vi "CAN Read Engine.vi"(6 "Current Scoket":i16, 8 "error in (no error)":errorcluster, 9 "Selected Sockets":i16[](array[numeric]), 10 "CAN Ref Out":refnum<class "NI-XNET.lvclass">[](array[class]), 11 "Notifier in":refnum<notifier>) -> (0 "error out":errorcluster)   [LabVIEW 2023, in "LTT_TeststandSteptypes.lvlib"]
uses:
  LTT_TeststandSteptypes.lvlib
  HardwareAbstractionLayer_LVOOP/CAN/CAN Lib/NI-XNET_class/NI-XNET.lvclass
  HardwareAbstractionLayer_LVOOP/CAN/CAN Lib/Control/CAN Table.ctl
  <vilib>/xnet/xnet.llb/XNET Frame CAN.ctl
  <vilib>/xnet/xnet.llb/XNET Frame Type CAN.ctl
  Control/CAN FGV State.ctl
  HardwareAbstractionLayer_LVOOP/Database/Database.lvclass
  HardwareAbstractionLayer_LVOOP/CAN/CAN Lib/CAN HAL Lib.lvlib
panel:
  in  "CAN View Table":T1=-1
  out "Read":bool
  out "Send":bool
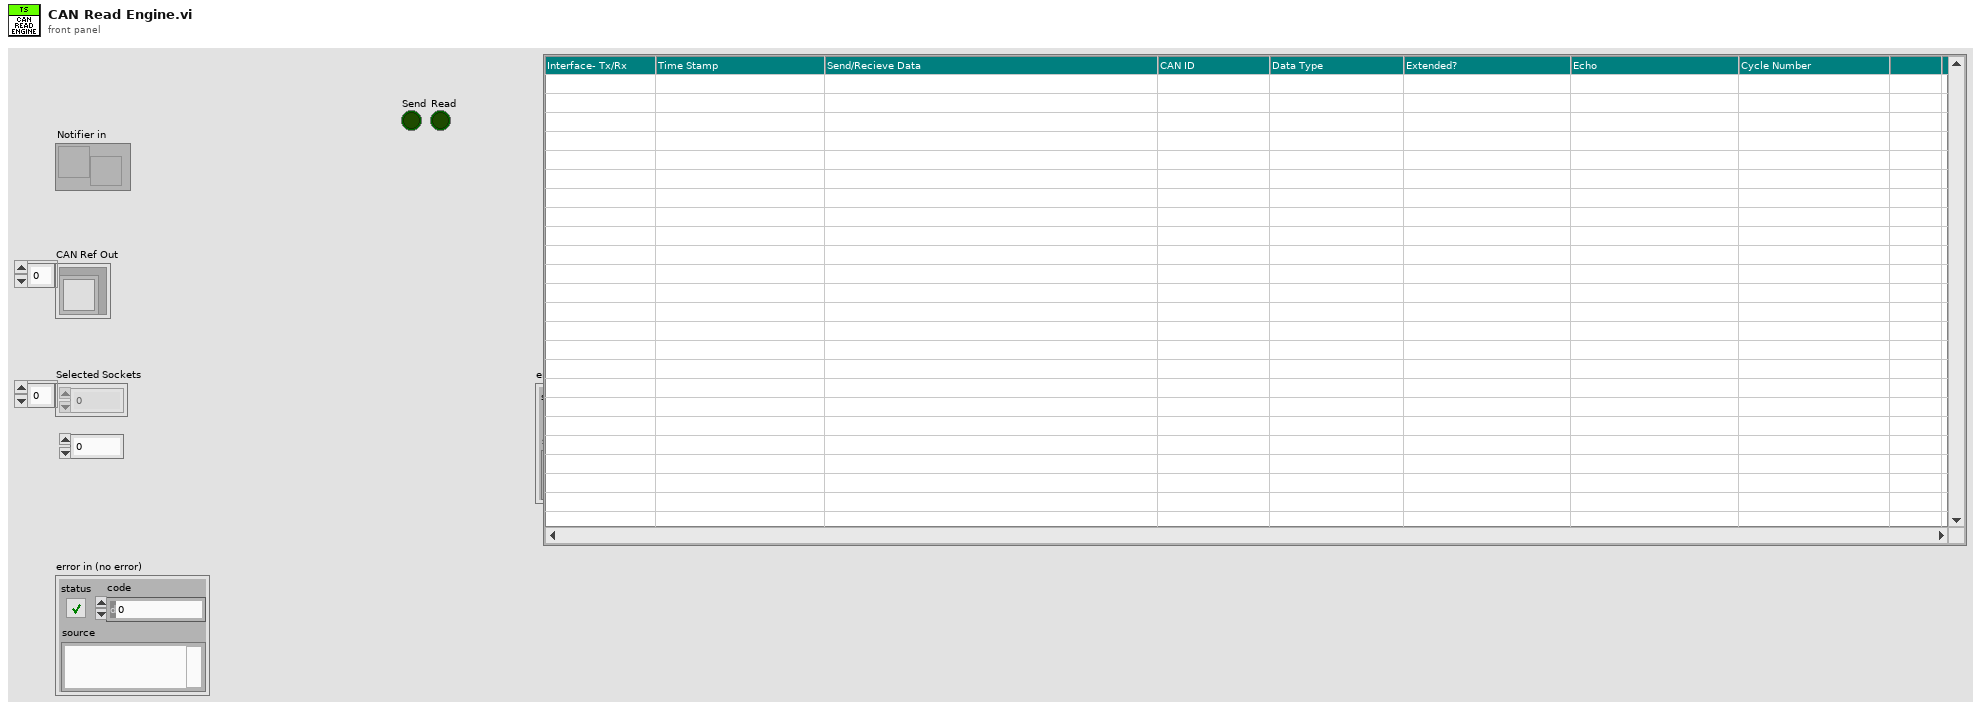
[diagram p1: front panel]
types:
  T1 = typedef "HardwareAbstractionLayer_LVOOP.lvlib/CAN HAL Lib.lvlib/CAN Table.ctl" = i32
  T2 = typedef "LTT_TeststandSteptypes.lvlib/CAN FGV State.ctl" = enum16{"Init", "Get", "Set"}
  T3 = typedef "XNET Frame CAN.ctl" = cluster{"timestamp":timestamp, "payload":u8[], "identifier":u32, "type":T4, "extended?":bool, "echo?":bool}
  T4 = typedef "XNET Frame Type CAN.ctl" = u8
  T5 = typedef "Semaphore RefNum" = refnum<k1>
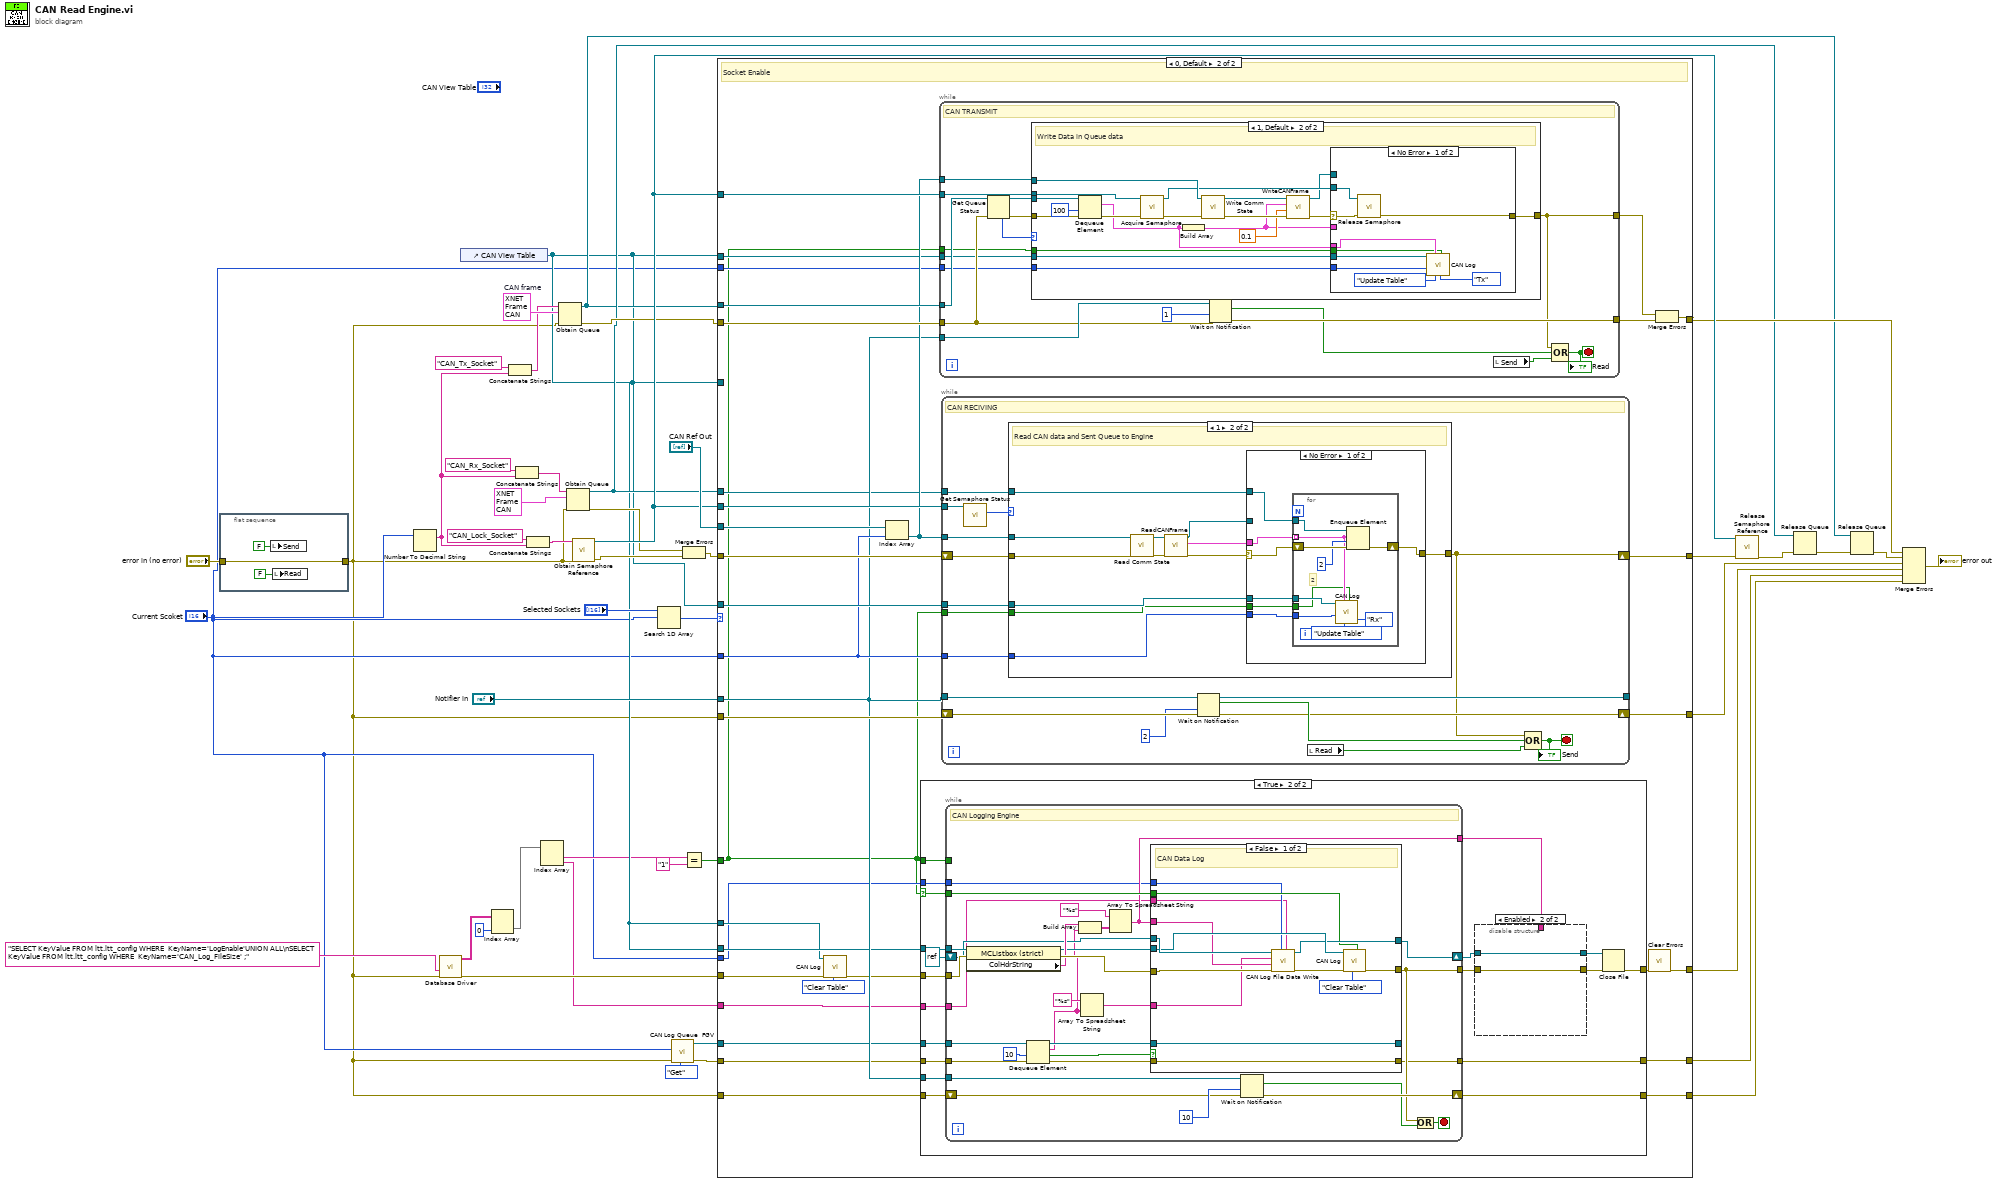
[diagram p0: block diagram]
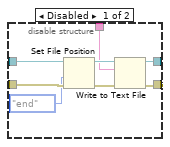
[diagram p4: hidden frame]
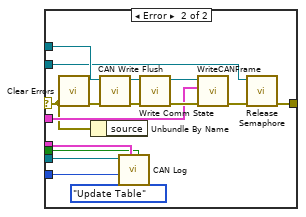
[diagram p7: hidden frame]
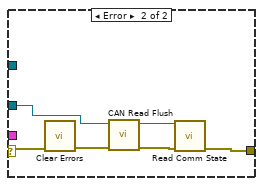
[diagram p9: hidden frame]
diagram:
  w35 = T3 {"timestamp"=timestamp(0 s since 1904-01-01), "payload"=[], "identifier"=0, "type"=0, "extended?"=FALSE, "echo?"=FALSE}  # CAN frame
  n1 = flat-sequence {
    tunnel: "error in (no error)" -> [w48]
    tunnel: [w48] -> w1
    frame #0 {
      n2 = local write "Send"(FALSE ("Send")) -> ()
      n3 = local write "Read"(FALSE ("Read")) -> ()
    }
  }
  n4 = Number To Decimal String(number="Current Scoket") -> (decimal integer string=w26:string)  [unwired: 1 in]
  n5 = call "Database Driver.vi"("error in"=w1, "SQL query"="SELECT KeyValue FROM ltt.ltt_config WHERE  KeyName='LogEnable'UNION ALL\nSELECT KeyValue FROM ltt.ltt_config WHERE  KeyName='CAN_Log_FileSize' ;") -> ("error out"=w10:errorcluster, "data"=w14:string[][])  [unwired: 6 in, 2 out]
  n6 = control-ref of="CAN View Table"() -> (w15:refnum<vi>)
  n7 = Index Array(array=w14, index (col)=0 ("disabled index (col)")) -> (element=w13:string[])  [unwired: 1 in]
  n8 = Concatenate Strings("CAN_Tx_Socket" ("name (unnamed)"), w26) -> (w32:string)
  n9 = Concatenate Strings("CAN_Rx_Socket" ("name (unnamed)"), w26) -> (w25:string)
  n10 = Concatenate Strings("CAN_Lock_Socket" ("name (unnamed)"), w26) -> (w38:string)
  n11 = Index Array(array=w13) -> (element #1=w8:string, element #2=w7:string)  [unwired: 2 in]
  n12 = Obtain Queue(name (unnamed)=w32, element data type=w35, error in (no error)=w1) -> (queue out=w17:refnum<queue>, error out=w34:errorcluster)  [unwired: 2 in, 1 out]
  n13 = Obtain Queue(name (unnamed)=w25, element data type=T3 {"timestamp"=timestamp(0 s since 1904-01-01), "payload"=[], "identifier"=0, "type"=0, "extended?"=FALSE, "echo?"=FALSE} ("CAN frame"), error in (no error)=w1) -> (queue out=w18:refnum<queue>, error out=w22:errorcluster)  [unwired: 2 in, 1 out]
  n14 = call <vilib>:"Obtain Semaphore Reference.vi"("error in (no error)"=w1, "name (unnamed)"=w38) -> ("error out"=w37:errorcluster, "semaphore"=w36:T5)  [unwired: 3 in, 1 out]
  n15 = Search 1D Array(1D array="Selected Sockets", element="Current Scoket") -> (index of element=w39:i32)  [unwired: 1 in]
  n16 = call "CAN Log Queue  FGV.vi"("CAN FGV State"=CAN_FGV_State."Get", "error in"=w1, "Current Scoket"="Current Scoket") -> ("error out"=w5:errorcluster, "Log queue out"=w3:refnum<queue>)  [unwired: 7 in]
  n17 = Merge Errors(w22, w37) -> (w23:errorcluster)
  n18 = Equal?(x=w8, y="1") -> (x = y?=w6:bool)
  n19 = case shown="0, Default" w39 {
    tunnel: [w55 w74] -> w46
    tunnel: w23 -> [w55 w86]
    tunnel: w36 -> [_ w89]
    tunnel: "Notifier in" -> [_ w72]
    tunnel: "CAN Ref Out" -> [_ w81]
    tunnel: w1 -> [w54 w88]
    tunnel: [w54 w87] -> w41
    tunnel: "Current Scoket" -> [_ w73]
    tunnel: w36 -> [_ w85]
    tunnel: w17 -> [_ w84]
    tunnel: w34 -> [w52 w83]
    tunnel: [w52 w79] -> w31
    tunnel: w15 -> [_ w75]
    tunnel: w15 -> [_ w77]
    tunnel: "Current Scoket" -> [_ w76]
    tunnel: w15 -> [_ _]
    tunnel: w10 -> [w53 w63]
    tunnel: w15 -> [_ w71]
    tunnel: [w53 w56] -> w30
    tunnel: w1 -> [w51 w69]
    tunnel: [w51 w68] -> w29
    tunnel: w18 -> [_ w67]
    tunnel: w5 -> [w50 w66]
    tunnel: w3 -> [_ w65]
    tunnel: [w50 w64] -> w16
    tunnel: "Current Scoket" -> [_ w59]
    tunnel: w15 -> [_ w62]
    tunnel: w7 -> [_ w58]
    tunnel: w6 -> [_ w57]
    frame -1 {
    }
    frame 0, Default {
      # "Socket Enable"
      n20 = call "CAN Log.vi"("Action"=enum16{"Update Table", "Clear Table"}."Clear Table", "error in (no error)"=w63, "CAN View Table"=w62) -> ("error out"=w60:errorcluster)  [unwired: 8 in]
      n21 = Index Array(array=w81, index=w73) -> (element=w80:refnum<class "NI-XNET.lvclass">)
      n22 = case shown="True" w57 {
        selector: w57 -> [_ w105]
        tunnel: w72 -> [_ w111]
        tunnel: w60 -> [w91 w110]
        tunnel: w71 -> [_ w109]
        tunnel: [w91 w108] -> w70
        tunnel: w69 -> [w92 w107]
        tunnel: [w92 w106] -> w68
        tunnel: w66 -> [w90 w99]
        tunnel: w65 -> [_ w98]
        tunnel: [w90 w97] -> w64
        tunnel: w59 -> [_ w96]
        tunnel: w57 -> [_ w95]
        tunnel: w58 -> [_ w94]
        frame False {
        }
        frame True {
          n23 = while {
            tunnel: w111 -> [w150]
            tunnel: w110 -> [w148]
            tunnel: w109 -> [w149]
            tunnel: [w136] -> w104
            shift-right: [w139] -> w106
            shift-left: w107 -> [w140]
            tunnel: w105 -> [w135]
            tunnel: [w134] -> w100
            tunnel: w99 -> [w132]
            tunnel: w98 -> [w133]
            tunnel: [w125] -> w97
            tunnel: w96 -> [w123]
            shift-right: [w141] -> w103
            shift-left: refnum<file> refnum ("Byte Stream File out") -> [w143]
            tunnel: w95 -> [_]
            tunnel: w94 -> [w122]
            stop <- w137 stop-if-true
            # "CAN Logging Engine"
            n24 = property class="MCListbox (strict)"(reference=w149, error in=w148) -> (reference out=w142:refnum<vi>, error out=w147:errorcluster, "ColHdrString"=w144:string[])
            n25 = Dequeue Element(queue=w133, timeout in ms (-1)=10, error in (no error)=w132) -> (queue out=w127:refnum<queue>, element=w124:string[], timed out?=w128:bool, error out=w126:errorcluster)
            n26 = Build Array(w144, w124) -> (w146:string[][])
            n27 = Array To Spreadsheet String(array=w124, 3:"%s" ("format string")) -> (spreadsheet string=w129:string)  [unwired: 1 in]
            n28 = Array To Spreadsheet String(array=w146, 3:"%s" ("format string")) -> (spreadsheet string=w134:string)  [unwired: 1 in]
            n29 = case shown="False" w128 {
              tunnel: w147 -> [w164 w168]
              tunnel: w143 -> [w165 w169]
              tunnel: w134 -> [w154 _]
              tunnel: w142 -> [w161 _]
              tunnel: [w160 w168] -> w136
              tunnel: [w159 w169] -> w141
              tunnel: w135 -> [w158 _]
              tunnel: w129 -> [w153 _]
              tunnel: w127 -> [w157 w167]
              tunnel: w126 -> [w156 w166]
              tunnel: [w157 w167] -> _
              tunnel: [w156 w166] -> w125
              tunnel: w123 -> [w155 _]
              tunnel: w122 -> [w152 _]
              frame False {
                # "CAN Data Log"
                n30 = call "CAN Log File Data Write.vi"("Size"=w152, "Socket"=w155, "error in (no error)"=w164, "With Column and CAN Data"=w154, "Without Column and CAN Data"=w153, "Byte Stream File in"=w165) -> ("error out"=w162:errorcluster, "Byte Stream File out"=w159:refnum<file>)  [unwired: 4 in]
                n31 = call "CAN Log.vi"("Log?"=w158, "Action"=enum16{"Update Table", "Clear Table"}."Clear Table", "error in (no error)"=w162, "CAN View Table"=w161) -> ("error out"=w160:errorcluster)  [unwired: 7 in]
              }
              frame True {
              }
            }
            n32 = Wait on Notification(notifier=w150, timeout in ms (-1)=10, error in (no error)=w140) -> (notification=w138:bool, error out=w139:errorcluster)  [unwired: 1 in, 2 out]
            n33 = Compound Arithmetic op=OR(w136, w138) -> (w137:bool)
          }
          n34 = disable-structure shown="Enabled" {
            disable-tunnel: w104 -> [w119 w120]
            disable-tunnel: w103 -> [w118 w121]
            disable-tunnel: [w116 w120] -> w102
            disable-tunnel: [w113 w121] -> w101
            disable-tunnel: w100 -> [w112 _]
            frame Disabled {
              n35 = Set File Position(refnum=w118, from (0:start)=enum16{"start", "end", "current"}."end", error in=w119) -> (refnum out=w115:refnum<file>, error out=w117:errorcluster)  [unwired: 1 in]
              n36 = Write to Text File(file (use dialog)=w115, text=w112, error in=w117) -> (refnum out=w113:refnum<file>, error out=w116:errorcluster)  [unwired: 1 in, 1 out]
            }
            frame Enabled {
            }
          }
          n37 = Close File(refnum=w101, error in=w102) -> (error out=w108:errorcluster)  [unwired: 1 out]
        }
      }
      n38 = while {
        tunnel: w72 -> [w186]
        tunnel: w85 -> [w183]
        tunnel: w84 -> [w179]
        tunnel: w83 -> [w181]
        tunnel: [w184] -> w82
        tunnel: w80 -> [w182]
        tunnel: [w173] -> w78
        tunnel: w77 -> [w172]
        tunnel: w76 -> [w171]
        tunnel: w57 -> [w170]
        stop <- w175 stop-if-true
        # "CAN TRANSMIT"
        n39 = Get Queue Status(queue=w179, error in (no error)=w181) -> (queue out=w178:refnum<queue>, error out=w180:errorcluster, # elements in queue=w177:i32)  [unwired: 1 in, 5 out]
        n40 = case shown="1, Default" w177 {
          tunnel: w183 -> [_ w205]
          tunnel: w182 -> [_ w204]
          tunnel: w180 -> [w187 w200]
          tunnel: w178 -> [_ w199]
          tunnel: [w187 w193] -> w173
          tunnel: w172 -> [_ w190]
          tunnel: w171 -> [_ w191]
          tunnel: w170 -> [_ w188]
          frame 0 {
            # "Queue is Emety"
          }
          frame 1, Default {
            # "Write Data in Queue data"
            n41 = Dequeue Element(queue=w199, timeout in ms (-1)=100, error in (no error)=w200) -> (element=w189:T3, error out=w206:errorcluster)  [unwired: 2 out]
            n42 = call <vilib>:"Acquire Semaphore.vi"("error in (no error)"=w206, "semaphore"=w205) -> ("error out"=w201:errorcluster, "semaphore out"=w195:T5)  [unwired: 3 in, 1 out]
            n43 = Build Array(w189) -> (w192:T3[])
            n44 = call-dynamic "Write Comm State.vi"("error in (no error)"=w201, "NI-XNET in"=w204) -> ("error out"=w198:errorcluster, "NI-XNET out"=w202:refnum<class "NI-XNET.lvclass">)  [unwired: 8 in]
            n45 = call-dynamic "WriteCANFrame.vi"("error in (no error)"=w198, "timeout (10)"=0.1, "data"=w192, "NI-XNET in"=w202) -> ("error out"=w196:errorcluster, "NI-XNET out"=w194:refnum<class "NI-XNET.lvclass">)  [unwired: 6 in]
            n46 = case shown="No Error" w196 {
              selector: w196 -> [w214 w216]
              tunnel: w195 -> [w215 w223]
              tunnel: w194 -> [_ w228]
              tunnel: [w213 w224] -> w193
              tunnel: w192 -> [_ w222]
              tunnel: w191 -> [w210 w217]
              tunnel: w190 -> [w209 w221]
              tunnel: w189 -> [w208 w220]
              tunnel: w188 -> [w207 w218]
              frame No Error {
                n47 = call <vilib>:"Release Semaphore.vi"("error in (no error)"=w214, "semaphore"=w215) -> ("error out"=w213:errorcluster)  [unwired: 4 in, 1 out]
                n48 = call "CAN Log.vi"("TX/RX?"=enum16{"Tx", "Rx"}."Tx", "Log?"=w207, "Action"=enum16{"Update Table", "Clear Table"}."Update Table", "CAN frame"=w208, "Socket No"=w210, "CAN View Table"=w209) -> ()  [unwired: 5 in, 1 out]
              }
              frame Error {
                n49 = call <vilib>:"Clear Errors.vi"("error in (no error)"=w216) -> ("error out"=w231:errorcluster)  [unwired: 5 in, 1 out]
                n50 = Unbundle By Name(w216) -> ()  [unwired: 1 out]
                n51 = call-dynamic "CAN Write Flush.vi"("error in (no error)"=w231, "NI-XNET in"=w228) -> ("error out"=w230:errorcluster, "NI-XNET out"=w227:refnum<class "NI-XNET.lvclass">)  [unwired: 8 in]
                n52 = call "CAN Log.vi"("Log?"=w218, "Action"=enum16{"Update Table", "Clear Table"}."Update Table", "CAN frame"=w220, "Socket No"=w217, "CAN View Table"=w221) -> ()  [unwired: 6 in, 1 out]
                n53 = call-dynamic "Write Comm State.vi"("error in (no error)"=w230, "NI-XNET in"=w227) -> ("error out"=w229:errorcluster, "NI-XNET out"=w226:refnum<class "NI-XNET.lvclass">)  [unwired: 8 in]
                n54 = call-dynamic "WriteCANFrame.vi"("error in (no error)"=w229, "data"=w222, "NI-XNET in"=w226) -> ("error out"=w225:errorcluster)  [unwired: 7 in, 1 out]
                n55 = call <vilib>:"Release Semaphore.vi"("error in (no error)"=w225, "semaphore"=w223) -> ("error out"=w224:errorcluster)  [unwired: 4 in, 1 out]
              }
            }
          }
        }
        n56 = Wait on Notification(notifier=w186, timeout in ms (-1)=1, error in (no error)=w181) -> (notification=w176:bool, error out=w184:errorcluster)  [unwired: 1 in, 2 out]
        n57 = local read "Send"() -> (w174:bool)
        n58 = Compound Arithmetic op=OR(w173, w176, w174) -> (w175:bool)
        "Read" <- w175
      }
      n59 = while {
        shift-right: [w234] -> w74
        shift-left: w86 -> [w241]
        tunnel: w72 -> [w248]
        tunnel: [w245] -> _
        shift-right: [w244] -> w87
        shift-left: w88 -> [w247]
        tunnel: w89 -> [w242]
        tunnel: w73 -> [w233]
        tunnel: w80 -> [w239]
        tunnel: w75 -> [w236]
        tunnel: w57 -> [w235]
        tunnel: w67 -> [w232]
        stop <- w238 stop-if-true
        # "CAN RECIVING"
        n60 = call <vilib>:"Get Semaphore Status.vi"("semaphore"=w242) -> ("# available"=w240:i32)  [unwired: 5 in, 5 out]
        n61 = case shown="1" w240 {
          tunnel: [w249 w251] -> w234
          tunnel: w241 -> [w249 w261]
          tunnel: w233 -> [_ w254]
          tunnel: w239 -> [_ w256]
          tunnel: w236 -> [_ w255]
          tunnel: w235 -> [_ w253]
          tunnel: w232 -> [_ w250]
          frame 0, Default {
            # "Queue is Emety"
          }
          frame 1 {
            # "Read CAN data and Sent Queue to Engine"
            n62 = call-dynamic "Read Comm State.vi"("error in (no error)"=w261, "NI-XNET in"=w256) -> ("error out"=w257:errorcluster, "NI-XNET out"=w258:refnum<class "NI-XNET.lvclass">)  [unwired: 8 in]
            n63 = call-dynamic "ReadCANFrame.vi"("error in (no error)"=w257, "NI-XNET in"=w258) -> ("error out"=w259:errorcluster, "data"=w260:T3[], "NI-XNET out"=w252:refnum<class "NI-XNET.lvclass">)  [unwired: 7 in]
            n64 = case shown="No Error" w259 {
              selector: w259 -> [w266 w281]
              tunnel: [w268 w279] -> w251
              tunnel: w260 -> [w267 _]
              tunnel: w255 -> [w265 _]
              tunnel: w254 -> [w264 _]
              tunnel: w253 -> [w263 _]
              tunnel: w252 -> [_ w280]
              tunnel: w250 -> [w262 _]
              frame No Error {
                n65 = for {
                  shift-right: [w277] -> w268
                  shift-left: w266 -> [w278]
                  tunnel: w267 -> [w275] mode=indexing
                  tunnel: w265 -> [w274]
                  tunnel: w264 -> [w271]
                  tunnel: w263 -> [w270]
                  tunnel: w262 -> [w269]
                  # "2"
                  n66 = call "CAN Log.vi"("TX/RX?"=enum16{"Tx", "Rx"}."Rx", "Log?"=w270, "Action"=enum16{"Update Table", "Clear Table"}."Update Table", "CAN frame"=w275, "Socket No"=w271, "CAN View Table"=w274) -> ()  [unwired: 5 in, 1 out]
                  n67 = Enqueue Element(queue=w269, element=w275, timeout in ms (-1)=2, error in (no error)=w278) -> (error out=w277:errorcluster)  [unwired: 2 out]
                }
              }
              frame Error {
                n68 = call <vilib>:"Clear Errors.vi"("error in (no error)"=w281) -> ("error out"=w284:errorcluster)  [unwired: 5 in, 1 out]
                n69 = call-dynamic "CAN Read Flush.vi"("error in (no error)"=w284, "NI-XNET in"=w280) -> ("error out"=w283:errorcluster, "NI-XNET out"=w282:refnum<class "NI-XNET.lvclass">)  [unwired: 8 in]
                n70 = call-dynamic "Read Comm State.vi"("error in (no error)"=w283, "NI-XNET in"=w282) -> ("error out"=w279:errorcluster)  [unwired: 8 in, 1 out]
              }
            }
          }
        }
        n71 = Wait on Notification(notifier=w248, timeout in ms (-1)=2, error in (no error)=w247) -> (notifier out=w245:refnum<notifier>, notification=w246:bool, error out=w244:errorcluster)  [unwired: 1 in, 1 out]
        n72 = local read "Read"() -> (w237:bool)
        n73 = Compound Arithmetic op=OR(w234, w246, w237) -> (w238:bool)
        "Send" <- w238
      }
      n74 = call <vilib>:"Clear Errors.vi"("error in (no error)"=w70) -> ("error out"=w56:errorcluster)  [unwired: 5 in, 1 out]
      n75 = Merge Errors(w78, w82) -> (w79:errorcluster)
    }
  }
  n76 = call <vilib>:"Release Semaphore Reference.vi"("error in (no error)"=w46, "semaphore"=w36) -> ("error out"=w21:errorcluster)  [unwired: 8 in, 1 out]
  n77 = Release Queue(queue=w18, error in (no error)=w21) -> (error out=w20:errorcluster)  [unwired: 1 in, 2 out]
  n78 = Release Queue(queue=w17, error in (no error)=w20) -> (error out=w19:errorcluster)  [unwired: 1 in, 2 out]
  n79 = Merge Errors(w31, w19, w41, w30, w16, w29) -> (→"error out":errorcluster)
